vi "LF Write File__ogtk.vi"   [LabVIEW 2012]
doc: "Writes data using a double precision number as offset to work for files larger than 2GB."
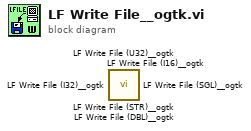
[diagram p0: block diagram]
diagram:
  n1 = call <userlib>:"LF Write File (STR)__ogtk.vi"() -> ()  [unwired: 8 in, 3 out]
  n2 = call <userlib>:"LF Write File (I16)__ogtk.vi"() -> ()  [unwired: 8 in, 3 out]
  n3 = call <userlib>:"LF Write File (I32)__ogtk.vi"() -> ()  [unwired: 8 in, 3 out]
  n4 = call <userlib>:"LF Write File (SGL)__ogtk.vi"() -> ()  [unwired: 8 in, 3 out]
  n5 = call <userlib>:"LF Write File (DBL)__ogtk.vi"() -> ()  [unwired: 8 in, 3 out]
  n6 = call <userlib>:"LF Write File (U32)__ogtk.vi"() -> ()  [unwired: 8 in, 3 out]
